vi "Oracle Popup.vi"(8 "error in":errorcluster) -> (0 "error out":errorcluster, 3 "SR array out":i32[](array[numeric]))   [LabVIEW 2018]
uses:
  <vilib>/Utility/miscctls.llb/LVPointTypeDef.ctl
panel:
  in  "Calling VI Refnum in":refnum<vi>
  in  "Ok Button":bool
  in  "Copied Text":string
  in  "Close":bool
  # "In your Universal Work Queue in Oracle, right-click anywhere in the table and select \"Copy All Rows.\" Paste the copied information in the string container below, then press \"OK\"."
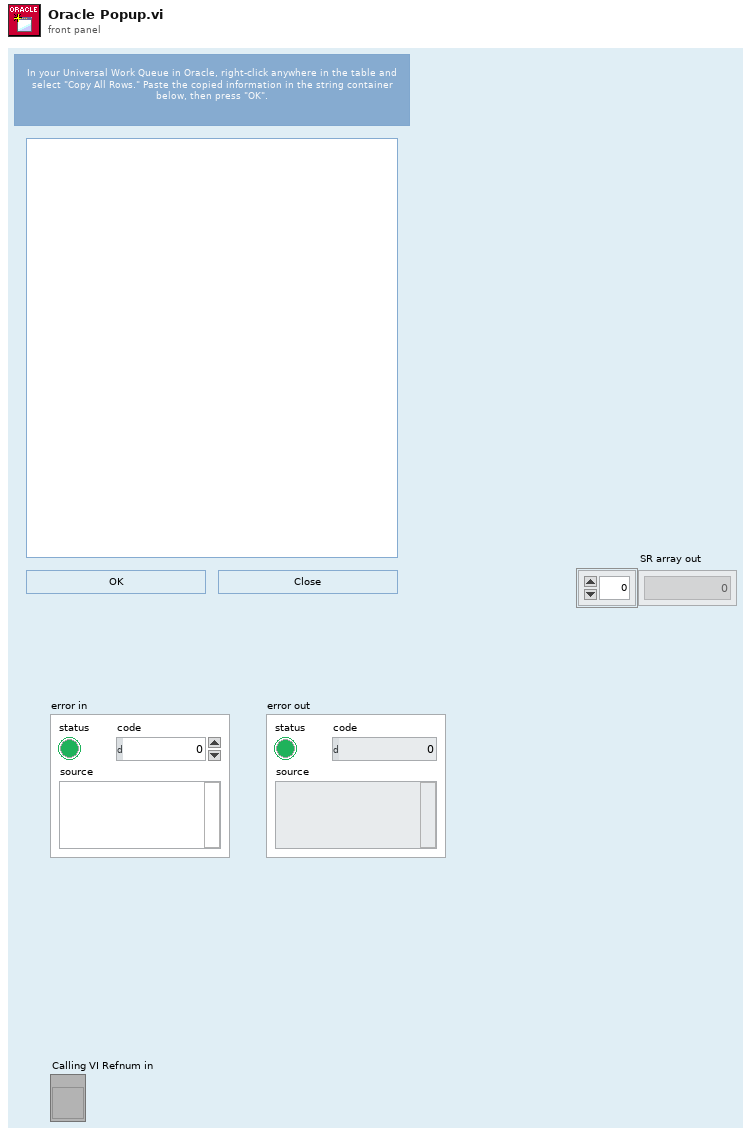
[diagram p1: front panel]
types:
  T1 = typedef "LVPointTypeDef.ctl" = cluster{"Horizontal":i16, "Vertical":i16}
  T2 = typedef "LVRectTypeDef.ctl" = cluster{"Left":i16, "Top":i16, "Right":i16, "Bottom":i16}
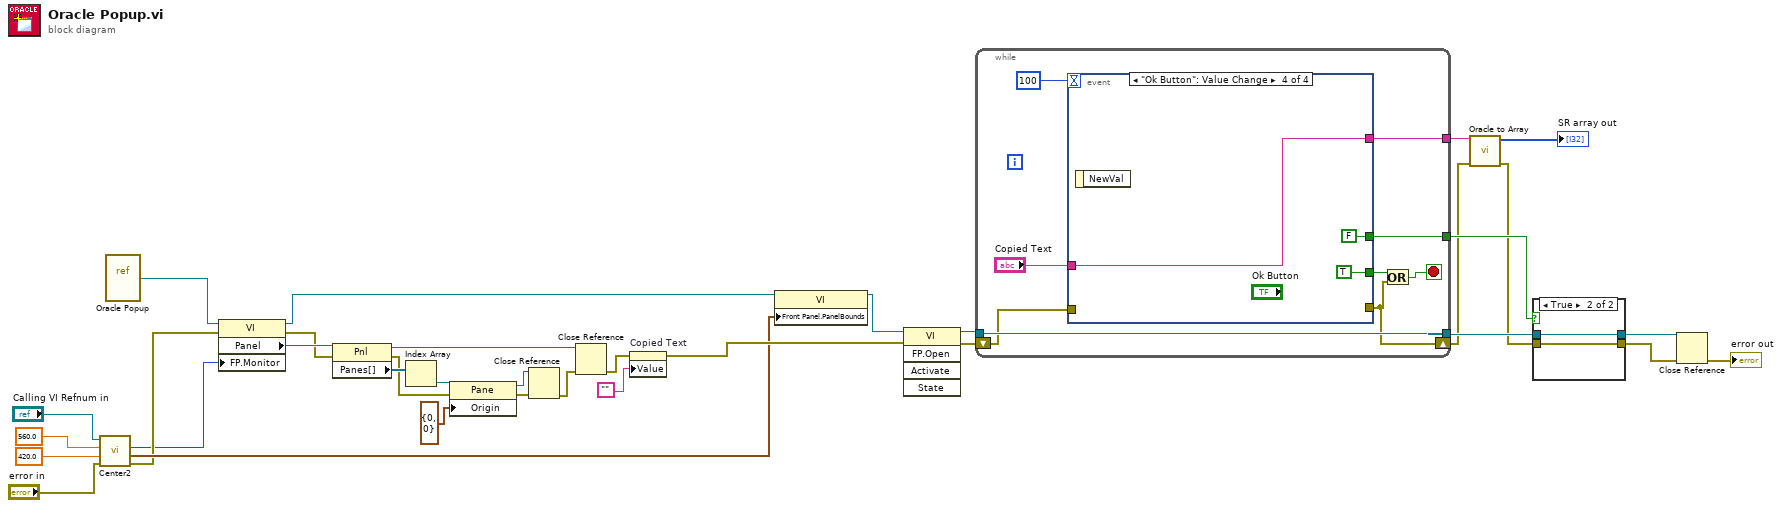
[diagram p0: block diagram]
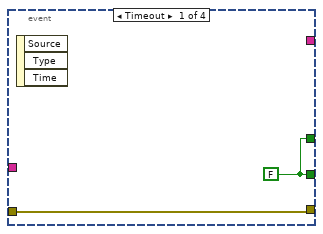
[diagram p2: hidden frame]
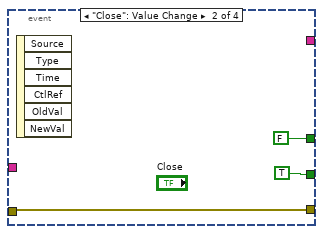
[diagram p3: hidden frame]
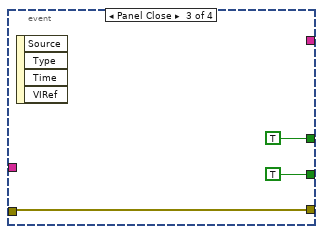
[diagram p4: hidden frame]
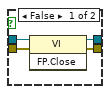
[diagram p5: hidden frame]
diagram:
  n1 = call "Center2.vi"("error in (no error)"="error in", "Width"=420.0, "Height"=560.0, "VI in"="Calling VI Refnum in") -> ("error out"=w9:errorcluster, "New Bounds"=w10:T2, "Active Monitor"=w5:u16)  [unwired: 5 in]
  n2 = vi-ref "Oracle Popup.vi"() -> (w31:refnum<vi>)
  n3 = property class="VI"(reference=w31, error in=w9, "FP.Monitor"=w5) -> (reference out=w12:refnum<vi>, error out=w21:errorcluster, "Panel"=w22:refnum<vi>)
  n4 = property class="Pnl"(reference=w22, error in=w21) -> (reference out=w23:refnum<vi>, error out=w28:errorcluster, "Panes[]"=w30:refnum<vi>[])
  n5 = Index Array(array=w30) -> (element=w29:refnum<vi>)  [unwired: 1 in]
  n6 = property class="Pane"(reference=w29, error in=w28, "Origin"=T1 {"Horizontal"=0, "Vertical"=0}) -> (reference out=w26:refnum<vi>, error out=w25:errorcluster)
  n7 = Close Reference(reference=w26, error in (no error)=w25) -> (error out=w24:errorcluster)
  n8 = Close Reference(reference=w23, error in (no error)=w24) -> (error out=w15:errorcluster)
  n9 = property on="Copied Text" class="Str"(error in=w15, "Value"="") -> (error out=w13:errorcluster)  [unwired: 1 in, 1 out]
  n10 = property class="VI"(reference=w12, "Front Panel.PanelBounds"=w10) -> (reference out=w11:refnum<vi>)  [unwired: 1 in, 1 out]
  n11 = invoke class="VI" method="FP.Open"(reference=w11, error in=w13) -> (reference out=w17:refnum<vi>, error out=w16:errorcluster)  [unwired: 3 in, 3 out]
  n12 = while {
    tunnel: [w43] -> w34
    tunnel: w17 -> [w43]
    shift-right: [w37] -> w2
    shift-left: w16 -> [w40]
    tunnel: [w36] -> w18
    tunnel: [w35] -> w4
    stop <- w38 stop-if-true
    n13 = event shown="[3] \"Ok Button\": Value Change" {
      selector: _ -> [_ _ _ _]
      dyn-events: _ -> [_ _ _ _]
      timeout: 100 -> [_ _ _ _]
      tunnel: [w44 TRUE ("Stop") TRUE ("Stop") TRUE ("Stop")] -> w39
      tunnel: "Copied Text" -> [_ _ _ w52]
      tunnel: w40 -> [w45 w47 w50 _]
      tunnel: [w45 w47 w50 _] -> w37
      tunnel: [w44 FALSE ("Stop") TRUE ("Stop") FALSE ("Stop")] -> w36
      tunnel: [_ _ _ w52] -> w35
      event Timeout {
        w44 = FALSE ("Stop")
        n14 = event-data() -> ()  [unwired: 1 in, 3 out]
      }
      event "Close": Value Change {
        n15 = event-data() -> ()  [unwired: 1 in, 6 out]
      }
      event Panel Close {
        n16 = event-data() -> ()  [unwired: 1 in, 4 out]
      }
      event "Ok Button": Value Change {
        n17 = event-data() -> ()  [unwired: 1 in, 1 out]
      }
    }
    n18 = Or(x=w39, y=w37) -> (x .or. y?=w38:bool)
  }
  n19 = call "Oracle to Array.vi"("error in"=w2, "string in"=w4) -> ("error out"=w1:errorcluster, "SR number array out"=→"SR array out":i32[])  [unwired: 7 in, 1 out]
  n20 = case shown="True" w18 {
    tunnel: w34 -> [w58 w60]
    tunnel: w1 -> [w57 w59]
    tunnel: [w56 w60] -> w33
    tunnel: [w55 w59] -> w32
    frame False {
      n21 = invoke class="VI" method="FP.Close"(reference=w58, error in=w57) -> (reference out=w56:refnum<vi>, error out=w55:errorcluster)  [unwired: 1 in, 1 out]
    }
    frame True {
    }
  }
  n22 = Close Reference(reference=w33, error in (no error)=w32) -> (error out=→"error out":errorcluster)
